vi "checkRepeat.vi"(11 "StringIN":string) -> (2 "StringOUT":string, 3 "NewString":bool)   [LabVIEW 2018, in "RunningLog.lvclass"]
uses:
  RunningLog.lvclass
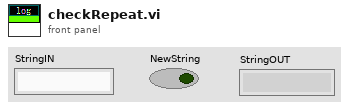
[diagram p1: front panel]
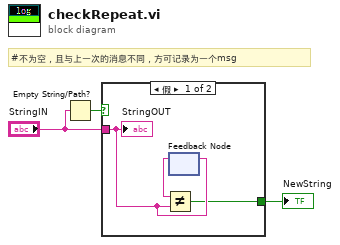
[diagram p0: block diagram]
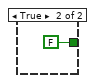
[diagram p2: hidden frame]
diagram:
  # "#不为空，且与上一次的消息不同，方可记录为一个msg"
  n1 = Empty String/Path?(string/path="StringIN") -> (empty?=w1:bool)
  n2 = case shown="假" w1 {
    tunnel: "StringIN" -> [w5 _]
    tunnel: [w4 FALSE] -> w2
    frame False {
      n3 = feedback #1() -> (w6:string)  [unwired: 1 in]
      n4 = Not Equal?(x=w6, y=w5) -> (x != y?=w4:bool)
      n5 = feedback-in #1(w5) -> ()
      "StringOUT" <- w5
    }
    frame True {
    }
  }
  "NewString" <- w2
